vi "Build CI URL.vi"(8 "error in":errorcluster, 11 "Parameters":variant) -> (0 "error out":errorcluster, 3 "Parameters out":variant)   [LabVIEW 2014, in "Jenkins Builder.lvclass"]
uses:
  Jenkins Builder.lvclass
  <vilib>/wsapi/NI_WebServices.lvlib
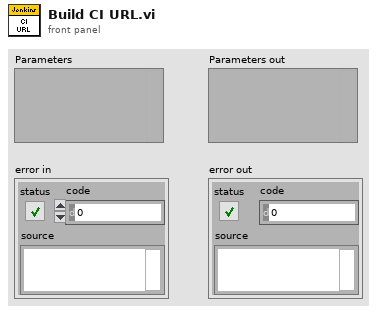
[diagram p1: front panel]
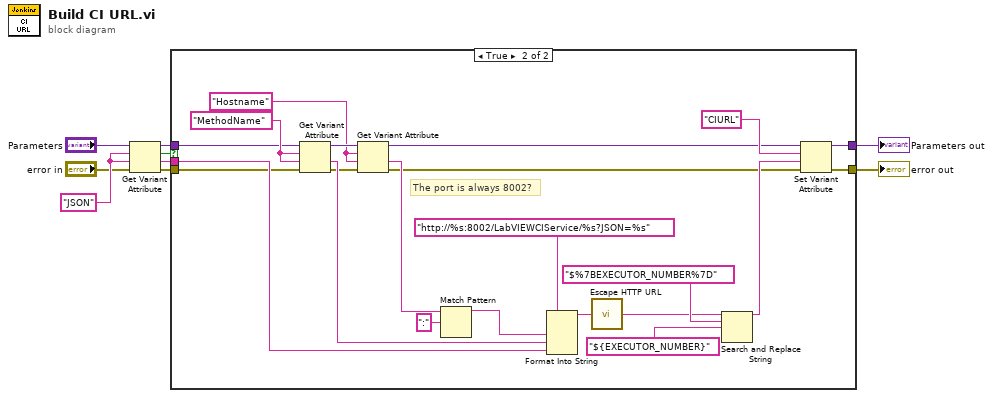
[diagram p0: block diagram]
diagram:
  w9 = "JSON" ("name")
  n1 = Get Variant Attribute(Variant="Parameters", name=w9, default value (empty Variant)=w9, error in="error in") -> (duplicate Variant=w7:variant, found=w1:bool, value=w8:string, error out=w4:errorcluster)
  n2 = case shown="True" w1 {
    tunnel: w8 -> [_ w24]
    tunnel: w7 -> [w11 w21]
    tunnel: [w11 w16] -> w5
    tunnel: w4 -> [w10 w15]
    tunnel: [w10 w12] -> w3
    frame False {
    }
    frame True {
      w19 = "Hostname" ("name")
      w22 = "MethodName" ("name")
      # "The port is always 8002?"
      n3 = Get Variant Attribute(Variant=w21, name=w22, default value (empty Variant)=w22, error in=w15) -> (duplicate Variant=w20:variant, value=w23:string, error out=w14:errorcluster)  [unwired: 1 out]
      n4 = Get Variant Attribute(Variant=w20, name=w19, default value (empty Variant)=w19, error in=w14) -> (duplicate Variant=w17:variant, value=w18:string, error out=w13:errorcluster)  [unwired: 1 out]
      n5 = Match Pattern(string=w18, regular expression=":") -> (before substring=w31:string)  [unwired: 1 in, 3 out]
      n6 = Format Into String(format string="http://%s:8002/LabVIEWCIService/%s?JSON=%s", w31, w23, w24) -> (resulting string=w30:string)  [unwired: 2 in, 1 out]
      n7 = call <vilib>:"Escape HTTP URL.vi"("unescaped string in"=w30) -> ("escaped string out"=w28:string)
      n8 = Search and Replace String(input string=w28, search string="$%7BEXECUTOR_NUMBER%7D" ("replace string (\"\")"), replace string="${EXECUTOR_NUMBER}" ("Executor_Number")) -> (result string=w26:string)  [unwired: 5 in, 3 out]
      n9 = Set Variant Attribute(Variant=w17, name="CIURL" ("Name"), value=w26, error in=w13) -> (Variant out=w16:variant, error out=w12:errorcluster)  [unwired: 1 out]
    }
  }
  "Parameters out" <- w5
  "error out" <- w3
